vi "SUB_ASKLEDS.vi"(1 "Pass Button":enum32{"No Selection", "Pass", "None"}(radio)=enum."Pass") -> ()   [LabVIEW 2011]
doc: "This is an example of how to use the radio buttons control with the Value Changed event."
panel:
  out "NewVal":enum32{"No Selection", "NG", "None"}(ring)
  in  "NG Button":enum32{"No Selection", "NG", "None"}(radio)=enum."NG"
  # "LEDS 有顯示正常?"
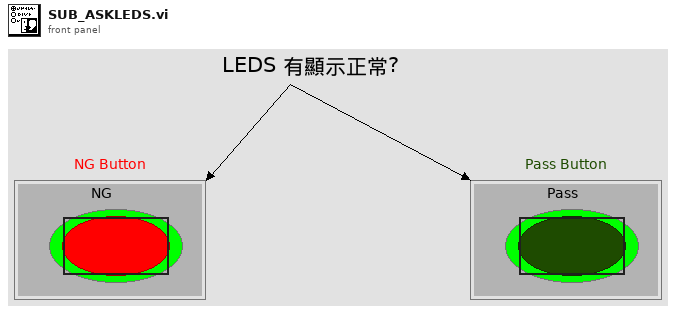
[diagram p1: front panel]
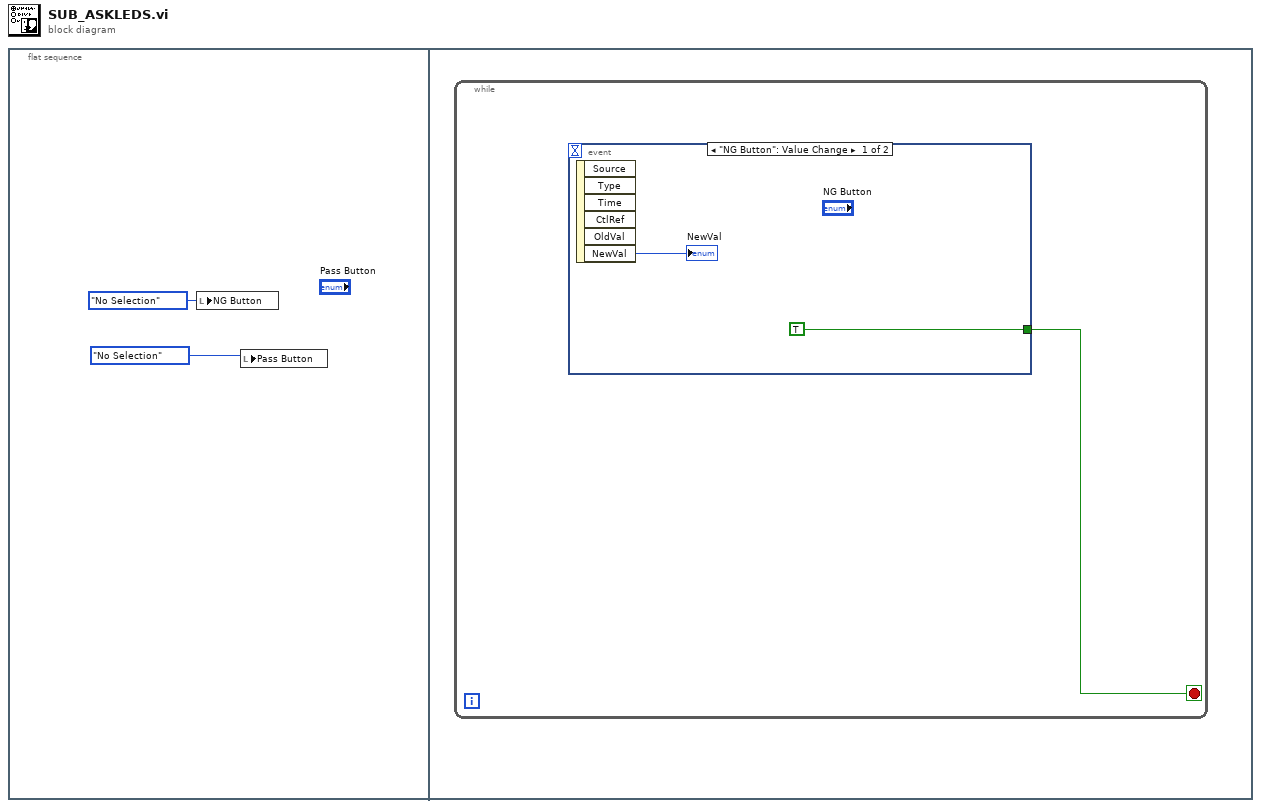
[diagram p0: block diagram]
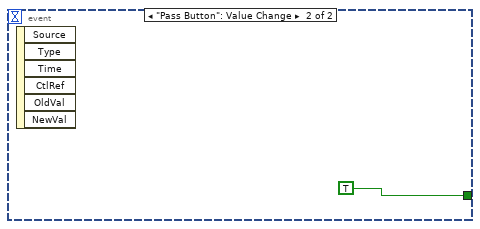
[diagram p2: hidden frame]
diagram:
  n1 = flat-sequence {
    frame #0 {
      n2 = local write "NG Button"(enum32{"No Selection", "NG", "None"}."No Selection" ("NG Button")) -> ()
      n3 = local write "Pass Button"(enum32{"No Selection", "Pass", "None"}."No Selection" ("Pass Button")) -> ()
    }
    frame #1 {
      n4 = while {
        stop <- w3 stop-if-true
        n5 = event shown="[0] \"NG Button\": Value Change" {
          selector: _ -> [_ _]
          dyn-events: _ -> [_ _]
          timeout: _ -> [_ _]
          tunnel: [TRUE TRUE] -> w3
          event "NG Button": Value Change {
            n6 = event-data() -> ("NewVal"=→"NewVal":enum32{"No Selection", "NG", "None"})  [unwired: 1 in, 5 out]
          }
          event "Pass Button": Value Change {
            n7 = event-data() -> ()  [unwired: 1 in, 6 out]
          }
        }
      }
    }
  }
